vi "OP500Z8P_ISOmicro.vi"(4 "reference":refnum<vi>, 6 "critere Iso":dbl, 8 "errin":errorcluster, 9 "Booléen":bool, 10 "Application Directory":path, 11 "VISA Refnum in":refnum<visa-resource-name>) -> (0 "error out":errorcluster, 2 "Ok ?":bool, 3 "String":string)   [LabVIEW 2020]
uses:
  C:/Users/elhajj/OneDrive - FORSEE POWER/Bureau/Support banc de test/Ligne ZENPLUS/Code LabVIEW/CODE/02 SLIM ZEN WS 500/SubVi/FGV.ctl
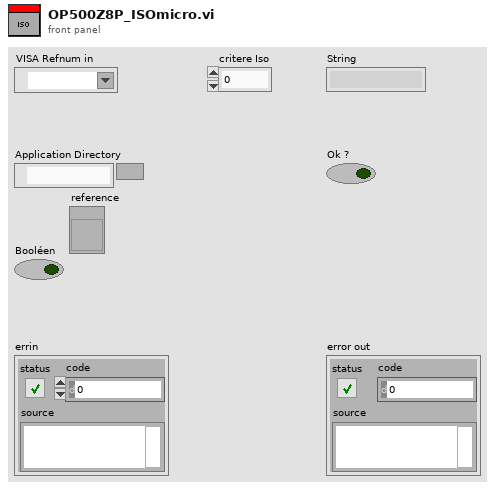
[diagram p1: front panel]
types:
  T1 = typedef "FGV.ctl" = enum16{"GET", "SET", "RAZ"}
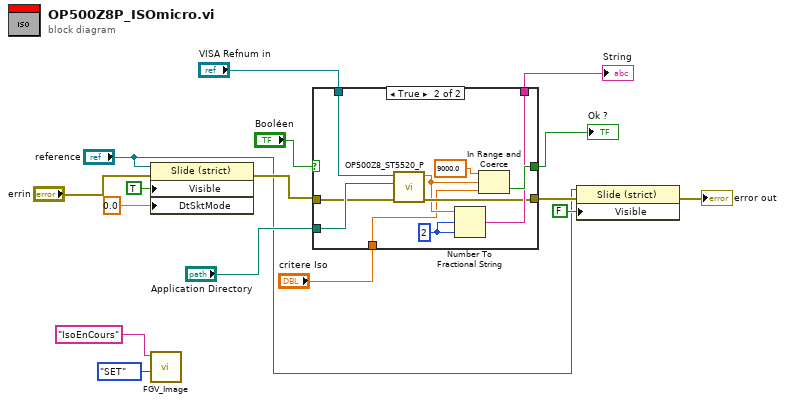
[diagram p0: block diagram]
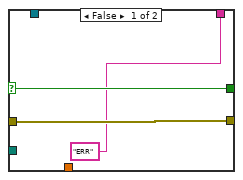
[diagram p2: hidden frame]
diagram:
  n1 = property on="Property Node" class="Slide (strict)"(reference="reference", error in="errin", "Visible"=TRUE ("Caption"), "DtSktMode"=0.0 ("DataSocket:Mode")) -> (error out=w9:errorcluster)  [unwired: 1 out]
  n2 = call "FGV_Image.vi"("Énum"=FGV."SET", "IN"="IsoEnCours") -> ()  [unwired: 9 in, 1 out]
  n3 = case shown="True" "Booléen" {
    selector: "Booléen" -> [w18 _]
    tunnel: w9 -> [w19 w25]
    tunnel: [w19 w24] -> w6
    tunnel: [w18 w28] -> w12
    tunnel: "critere Iso" -> [_ w20]
    tunnel: ["ERR" w27] -> w11
    tunnel: "Application Directory" -> [_ w26]
    tunnel: "VISA Refnum in" -> [_ w23]
    frame False {
    }
    frame True {
      w29 = i16 2 ("largeur (-)")
      n4 = call "OP500Z8_ST5520_P.vi"("errin"=w25, "chemin de base"=w26, "Refnum VISA en entrée"=w23) -> ("error out"=w24:errorcluster, "R iso(MOhm)"=w22:dbl)  [unwired: 7 in]
      n5 = Number To Fractional String(number=w22, width (-)=w29, precision (6)=w29) -> (F-format string=w27:string)  [unwired: 1 in]
      n6 = In Range and Coerce(upper limit=9000.0 ("limite supérieure"), x=w22, lower limit=w20) -> (In Range?=w28:bool)  [unwired: 1 out]
    }
  }
  "Ok ?" <- w12
  "String" <- w11
  n7 = property on="Property Node" class="Slide (strict)"(reference="reference", error in=w6, "Visible"=FALSE ("Caption")) -> (error out=→"error out":errorcluster)  [unwired: 1 out]
